vi "PathPlanner_PathFinder_Heuristic.vi"(9 "sGoal":T1, 11 "sStart":T1) -> (3 "heuristic":dbl)   [LabVIEW 2019, in "PathPlanner24.lvlib"]
uses:
  PathPlanner24.lvlib
  TypeDef/PathPlannerFinderGridPosition.ctl
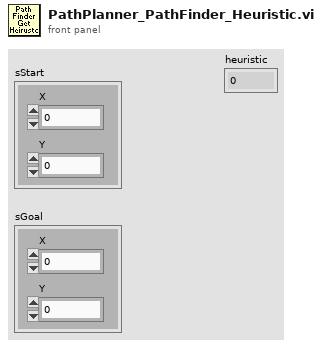
[diagram p1: front panel]
types:
  T1 = typedef "PathPlanner24.lvlib/PathPlannerFinderGridPosition.ctl" = cluster{"X":i32, "Y":i32}
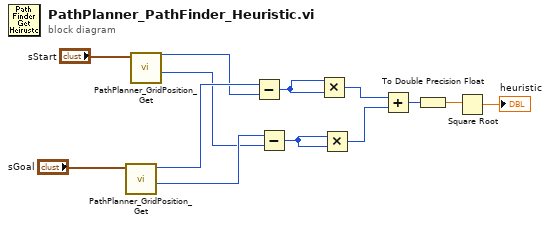
[diagram p0: block diagram]
diagram:
  n1 = call "PathPlanner_GridPosition_Get.vi"("GridPosition"="sGoal") -> ("Y"=w9:i32, "X"=w11:i32)  [unwired: 9 in]
  n2 = call "PathPlanner_GridPosition_Get.vi"("GridPosition"="sStart") -> ("Y"=w8:i32, "X"=w10:i32)  [unwired: 9 in]
  n3 = Subtract(x=w11, y=w10) -> (x-y=w7:i32)
  n4 = Subtract(x=w9, y=w8) -> (x-y=w6:i32)
  n5 = Multiply(x=w7, y=w7) -> (x*y=w4:i32)
  n6 = Multiply(x=w6, y=w6) -> (x*y=w3:i32)
  n7 = Add(x=w4, y=w3) -> (x+y=w5:i32)
  n8 = To Double Precision Float(number=w5) -> (double precision float=w2:dbl)
  n9 = Square Root(x=w2) -> (sqrt(x)=→"heuristic":dbl)
